vi "PH_Powermeter_BaseClass.set GUI Elements for the first time.vi"(0 "i ref in":refnum<vi>, 5 "error in":errorcluster) -> (14 "i ref out":refnum<vi>, 19 "error out":errorcluster)   [LabVIEW 2014, in "PH_Powermeter_BaseClass.lvlib"]
doc: "This VI indicates the wanted Settings at the GUI element."
uses:
  PH_Powermeter_BaseClass.lvlib
  PH_Common/PH_Common.lvlib
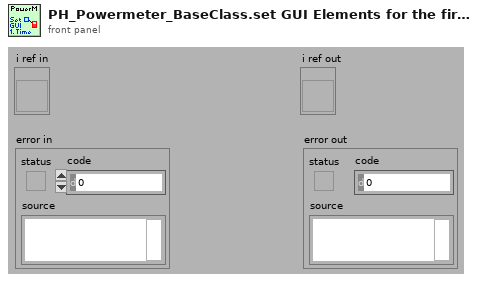
[diagram p1: front panel]
types:
  T1 = typedef "PH_Powermeter_BaseClass.lvlib/PH_Powermeter_BaseClass.i attribute.ctl" = cluster{"GUI References":T2, "Connection":T3, "Head Attributes":T5, "VISA resource":refnum<visa-resource-name>, "Energy":T6, "Service ID Energy":i32, "Wanted Settings":T7, "Current Settings":T7}
  T2 = typedef "PH_Powermeter_BaseClass.lvlib/PH_Powermeter_BaseClass.GUI Refs.ctl" = cluster{"Head Attributes":refnum<vi>, "Energy":refnum<vi>, "Connection":refnum<vi>, "VISA Resource":refnum<vi>, "Scaling Factor":refnum<vi>, "Range":refnum<vi>, "Wavelength":refnum<vi>, "Trigger Level":refnum<vi>, "Wanted Settings":refnum<vi>, "Current Settings":refnum<vi>}
  T3 = typedef "PH_Powermeter_BaseClass.lvlib/PH_Powermeter_BaseClass.Connection.ctl" = cluster{"failed checks":i8, "Timeout":bool, "Data read":string, "Failure":bool, "Error":bool, "State":T4}
  T4 = typedef "PH_Powermeter_BaseClass.lvlib/PH_Powermeter_BaseClass.State.ctl" = enum32{"off", "operating", "opened", "checked", "connected", "Sets to change", "running"}
  T5 = typedef "PH_Powermeter_BaseClass.lvlib/PH_Powermeter_BaseClass.Head Attributes.ctl" = cluster{"Instrument Type":string, "Head Version":string, "Head Name":string, "Serial Number":string, "Firmware":string, "Sensor Type":string, "MinimumRange":u32, "Maximum Range":u32, "Min Wavelength":i32, "Max Wavelength":i32}
  T6 = typedef "PH_Powermeter_BaseClass.lvlib/PH_Powermeter_BaseClass.Energy.ctl" = cluster{"current Value":dbl, "unscaled":dbl, "Scaling Factor":dbl}
  T7 = typedef "PH_Powermeter_BaseClass.lvlib/PH_gentec_BaseClass.Head Settings.ctl" = cluster{"Trigger Level":dbl, "Wavelength":u32, "Range":u32}
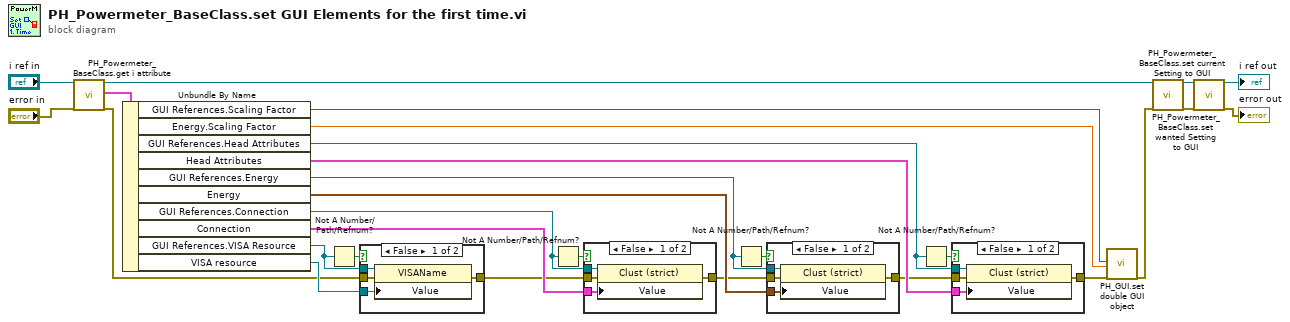
[diagram p0: block diagram]
diagram:
  n1 = call "PH_Powermeter_BaseClass.get i attribute.vi"("i ref in"="i ref in", "error in (no error)"="error in") -> ("i ref out"=w26:refnum<vi>, "i attribute"=w27:T1, "error out"=w17:errorcluster)  [unwired: 15 in]
  n2 = Unbundle By Name(w27) -> ("GUI References.Scaling Factor"=w7:refnum<vi>, "Energy.Scaling Factor"=w8:dbl, "GUI References.Head Attributes"=w21:refnum<vi>, "Head Attributes"=w23:T5, "GUI References.Energy"=w12:refnum<vi>, "Energy"=w11:T6, "GUI References.Connection"=w15:refnum<vi>, "Connection"=w14:T3, "GUI References.VISA Resource"=w19:refnum<vi>, "VISA resource"=w18:refnum<visa-resource-name>)
  n3 = Not A Number/Path/Refnum?(number/path/refnum=w19) -> (NaN/Path/Refnum?=w20:bool)
  n4 = case shown="False" w20 {
    tunnel: [w32 w33] -> w6
    tunnel: w19 -> [w31 _]
    tunnel: w17 -> [w30 w33]
    tunnel: w18 -> [w29 _]
    frame False {
      n5 = property class="VISAName"(reference=w31, error in=w30, "Value"=w29) -> (error out=w32:errorcluster)  [unwired: 1 out]
    }
    frame True {
    }
  }
  n6 = Not A Number/Path/Refnum?(number/path/refnum=w15) -> (NaN/Path/Refnum?=w16:bool)
  n7 = case shown="False" w16 {
    tunnel: [w37 w38] -> w10
    tunnel: w15 -> [w36 _]
    tunnel: w6 -> [w35 w38]
    tunnel: w14 -> [w34 _]
    frame False {
      n8 = property class="Clust (strict)"(reference=w36, error in=w35, "Value"=w34) -> (error out=w37:errorcluster)  [unwired: 1 out]
    }
    frame True {
    }
  }
  n9 = Not A Number/Path/Refnum?(number/path/refnum=w12) -> (NaN/Path/Refnum?=w13:bool)
  n10 = case shown="False" w13 {
    tunnel: [w42 w43] -> w9
    tunnel: w12 -> [w41 _]
    tunnel: w10 -> [w40 w43]
    tunnel: w11 -> [w39 _]
    frame False {
      n11 = property class="Clust (strict)"(reference=w41, error in=w40, "Value"=w39) -> (error out=w42:errorcluster)  [unwired: 1 out]
    }
    frame True {
    }
  }
  n12 = Not A Number/Path/Refnum?(number/path/refnum=w21) -> (NaN/Path/Refnum?=w22:bool)
  n13 = case shown="False" w22 {
    tunnel: [w47 w48] -> w28
    tunnel: w21 -> [w46 _]
    tunnel: w9 -> [w45 w48]
    tunnel: w23 -> [w44 _]
    frame False {
      n14 = property class="Clust (strict)"(reference=w46, error in=w45, "Value"=w44) -> (error out=w47:errorcluster)  [unwired: 1 out]
    }
    frame True {
    }
  }
  n15 = call "PH_GUI.set double GUI object.vi"("GUI object Ref"=w7, "value"=w8, "error in (no error)"=w28) -> ("error out"=w5:errorcluster)  [unwired: 16 in]
  n16 = call "PH_Powermeter_BaseClass.set wanted Setting to GUI.vi"("VI in"=w26, "error in (no error)"=w5) -> ("VI out"=w3:refnum<vi>, "error out"=w4:errorcluster)  [unwired: 16 in]
  n17 = call "PH_Powermeter_BaseClass.set current Setting to GUI.vi"("VI in"=w3, "error in (no error)"=w4) -> ("VI out"=→"i ref out":refnum<vi>, "error out"=→"error out":errorcluster)  [unwired: 16 in]
